vi "Step Flow.vi"(8 "error in (no error)":errorcluster, 11 "Wait On Boolean Step in":refnum<class "Wait On Boolean Step.lvclass">) -> (0 "error out":errorcluster, 3 "Wait On Boolean Step out":refnum<class "Wait On Boolean Step.lvclass">)   [LabVIEW 2015, in "Wait On Boolean Step.lvclass"]
uses:
  Wait On Boolean Step.lvclass
  classes/Step/Execution/StepState.ctl
  classes/Step/Execution/Step Status.ctl
  classes/Step/Execution/Step Flow Control.ctl
  Wait On Boolean Step.lvclass/Wait On Boolean Step.ctl
  classes/Step/Execution/Step.lvclass
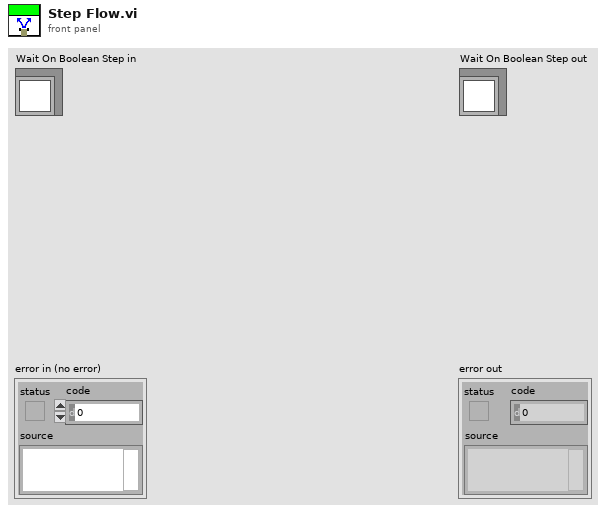
[diagram p1: front panel]
types:
  T1 = typedef "Step.lvclass/StepState.ctl" = cluster{"Step State":T2, "Flow Control":T3, "Jump Index":i32, "Done":bool}
  T2 = typedef "Step.lvclass/Step Status.ctl" = enum16{"Start", "Passed", "Failed", "Error", "Done", "Terminated", "Skipped", "Running"}
  T3 = typedef "Step.lvclass/Step Flow Control.ctl" = enum16{"Next Step", "Jump"}
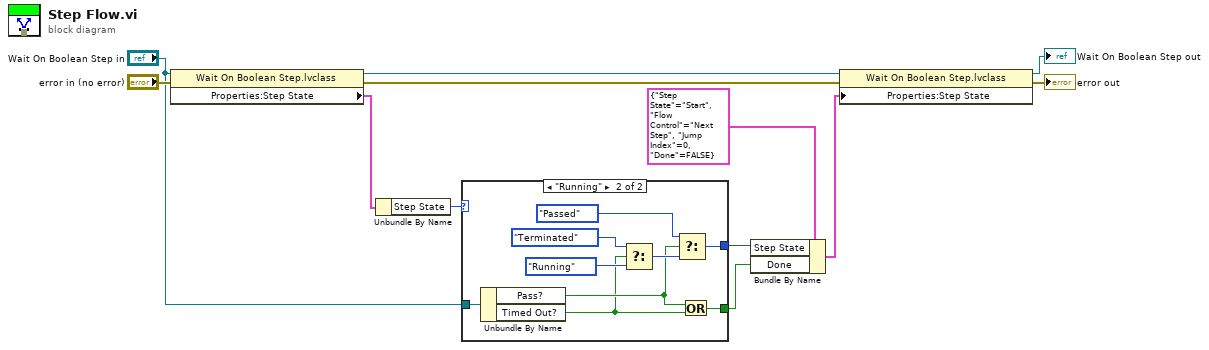
[diagram p0: block diagram]
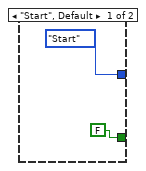
[diagram p2: hidden frame]
diagram:
  n1 = property class="Wait On Boolean Step.lvclass"(reference="Wait On Boolean Step in", error in="error in (no error)") -> (reference out=w7:refnum<class "Wait On Boolean Step.lvclass">, error out=w8:errorcluster, "Properties:Step State"=w10:T1)
  n2 = Unbundle By Name(w10) -> ("Step State"=w6:T2)
  n3 = case shown="\"Running\"" w6 {
    tunnel: "Wait On Boolean Step in" -> [_ w23]
    tunnel: [Step_Status."Start" ("Step State") w18] -> w3
    tunnel: [FALSE ("Done") w17] -> w1
    frame "Start", Default {
    }
    frame "Running" {
      n4 = Unbundle By Name(w23) -> ("Pass?"=w16:bool, "Timed Out?"=w15:bool)
      n5 = Select(t=Step_Status."Terminated", s=w15, f=Step_Status."Running" ("Step State")) -> (s? t:f=w20:T2)
      n6 = Select(t=Step_Status."Passed", s=w16, f=w20) -> (s? t:f=w18:T2)
      n7 = Or(x=w16, y=w15) -> (x .or. y?=w17:bool)
    }
  }
  n8 = Bundle By Name(cluster=T1 {"Step State"=enum."Start", "Flow Control"=enum."Next Step", "Jump Index"=0, "Done"=FALSE} ("Step State"), "Step State"=w3, "Done"=w1) -> (w2:T1)
  n9 = property class="Wait On Boolean Step.lvclass"(reference=w7, error in=w8, "Properties:Step State"=w2) -> (reference out=→"Wait On Boolean Step out":refnum<class "Wait On Boolean Step.lvclass">, error out=→"error out":errorcluster)
